vi "MB Param redefine.vi"(6 "conninfo":T1={"host"="localhost", "port"="5432", "client_encoding"="WIN1251", "dbname"="data", "user"="postgres", "password"=""}, 8 "error in (no error)":errorcluster, 9 "KFMTable":string="kfm_3", 10 "KFM param":string[](array[string]), 11 "MBs":refnum<class "Master CR.lvclass">[](array[class])) -> (0 "error":errorcluster, 3 "MBs out":refnum<class "Master CR.lvclass">[](array[class]))   [LabVIEW 2021]
uses:
  PostgreSQL/PostgreSQL2LabVIEW/ctl/Coninfo.ctl
  Master CR.lvclass
  TCP Param/Typedefs/KFMParamColumns.ctl
  TCP Param/TCP Param.lvclass
  D:/my_projects/projects/Algorithms/Labview/21/Master CR/Param/Param.lvclass
  Master CR.lvclass/Master CR.ctl
  Param.lvclass/Param.ctl
  TCP Param/TCP Param.lvclass/TCP Param.ctl
  Param.lvclass
  PostgreSQL/PostgreSQL2LabVIEW/libpqUtility/libpqutility.lvlib
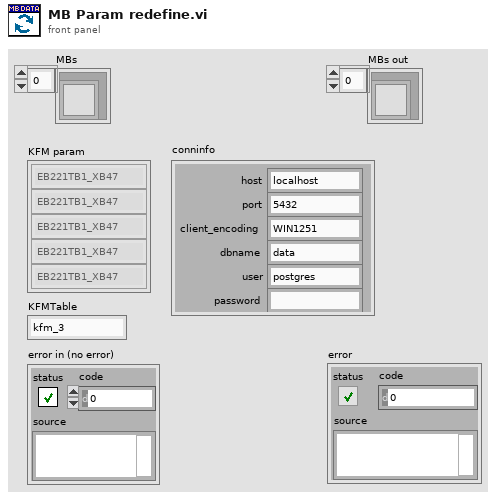
[diagram p1: front panel]
types:
  T1 = typedef "libpqutility.lvlib/Coninfo.ctl" = cluster{"host":string, "port":string, "client_encoding":string, "dbname":string, "user":string, "password":string}
  T2 = typedef "Param.lvlib/TCP Param.lvclass/KFMParamColumns.ctl" = enum16{"MVIName", "ip_adress", "port", "connection_timeout", "reconnection_timeout", "n_attempt_max", "reset_connect_timeout", "write_timeout", "read_timeout", "period", "enable", "write_enable", "fcode_full"}
  T3 = typedef "Param.lvlib/TCP Param.lvclass/timeouts.ctl" = cluster{"conn_timeout":i32, "reconn_timeout":i32, "N attempt max":i32, "t_reset_TTL":i32, "write_timeout":i32, "read_timeout":i32, "period":i32}
  T4 = cluster{"Remote IP Address":string, "Remote Port":u16}[]
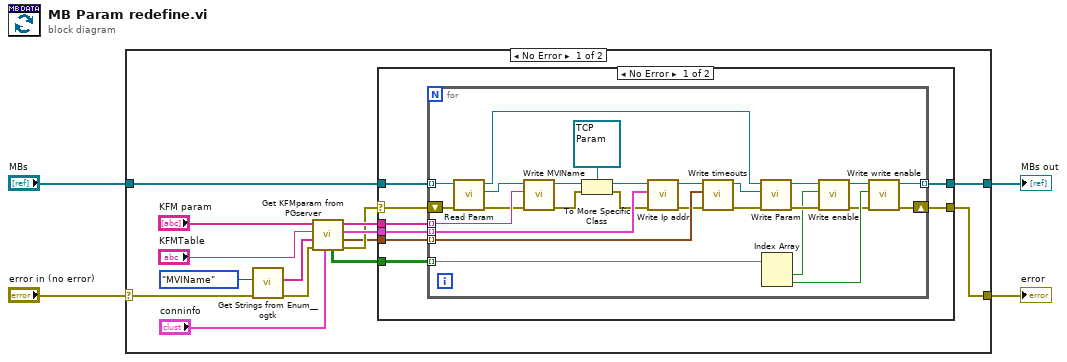
[diagram p0: block diagram]
diagram:
  n1 = case shown="No Error" "error in (no error)" {
    selector: "error in (no error)" -> [w9 w57]
    tunnel: [w19 w57] -> w4
    tunnel: "MBs" -> [w7 w56]
    tunnel: [w6 w56] -> w1
    frame No Error {
      n2 = call <userlib>:"Get Strings from Enum__ogtk.vi"("error in (no error)"=w9, "Enum"=KFMParamColumns."MVIName" ("KFMParamColumns")) -> ("error out"=w8:errorcluster, "Enum Strings"=w10:string[])  [unwired: 6 in, 2 out]
      n3 = call "Get KFMparam from PGserver.vi"("conninfo"="conninfo", "error in (no error)"=w8, "KFMParamColumns"=w10, "KFMParamTable"="KFMTable", "KFMParameters"="KFM param") -> ("error out"=w15:errorcluster, "timeouts"=w12:T3[], "IP Address"=w16:T4, "MVIName"=w17:string[], "enable"=w11:bool[][])  [unwired: 2 in]
      n4 = case shown="No Error" w15 {
        selector: w15 -> [w26 w55]
        tunnel: w17 -> [w23 _]
        tunnel: w16 -> [w25 _]
        tunnel: [w20 w55] -> w19
        tunnel: w12 -> [w24 _]
        tunnel: w11 -> [w22 _]
        tunnel: w7 -> [w27 w54]
        tunnel: [w21 w54] -> w6
        frame No Error {
          n5 = for {
            tunnel: w27 -> [w28] mode=indexing
            tunnel: w25 -> [w35] mode=indexing
            tunnel: w24 -> [w32] mode=indexing
            tunnel: w23 -> [w50] mode=indexing
            tunnel: w22 -> [w44] mode=indexing
            tunnel: [w40] -> w21 mode=indexing
            shift-right: [w39] -> w20
            shift-left: w26 -> [w53]
            n6 = call "Read Param.vi"("error in (no error)"=w53, "MB_TCP in"=w28) -> ("error out"=w48:errorcluster, "Param"=w51:refnum<class "Param.lvclass">, "MB_TCP out"=w47:refnum<class "Master CR.lvclass">)  [unwired: 7 in]
            n7 = call "Write MVIName.vi"("error in (no error)"=w48, "MVIName"=w50, "MB Param in"=w51) -> ("error out"=w37:errorcluster, "MB Param out"=w49:refnum<class "Param.lvclass">)  [unwired: 7 in]
            n8 = To More Specific Class(target class=refnum<class "TCP Param.lvclass"> refnum ("Param.lvlib:TCP Param.lvclass"), reference=w49, error in=w37) -> (specific class reference=w36:refnum<class "TCP Param.lvclass">, error out=w34:errorcluster)
            n9 = call "Write Ip addr.vi"("error in (no error)"=w34, "IP address"=w35, "MB Param in"=w36) -> ("error out"=w31:errorcluster, "MB Param out"=w33:refnum<class "TCP Param.lvclass">)  [unwired: 7 in]
            n10 = call "Write timeouts.vi"("error in (no error)"=w31, "timeouts"=w32, "MB Param in"=w33) -> ("error out"=w30:errorcluster, "MB Param out"=w29:refnum<class "TCP Param.lvclass">)  [unwired: 7 in]
            n11 = call "Write Param.vi"("error in (no error)"=w30, "Param"=w29, "MB_TCP in"=w47) -> ("error out"=w45:errorcluster, "MB_TCP out"=w46:refnum<class "Master CR.lvclass">)  [unwired: 7 in]
            n12 = Index Array(array=w44) -> (element #1=w43:bool, element #2=w42:bool)  [unwired: 2 in]
            n13 = call "Write enable.vi"("error in (no error)"=w45, "enable"=w43, "Master CR in"=w46) -> ("error out"=w41:errorcluster, "Master CR out"=w52:refnum<class "Master CR.lvclass">)  [unwired: 7 in]
            n14 = call "Write write enable.vi"("error in (no error)"=w41, "write enable"=w42, "Master CR in"=w52) -> ("error out"=w39:errorcluster, "Master CR out"=w40:refnum<class "Master CR.lvclass">)  [unwired: 7 in]
          }
        }
        frame Error {
        }
      }
    }
    frame Error {
    }
  }
  "error" <- w4
  "MBs out" <- w1
